vi "temp control global variables.vi"() -> ()   [LabVIEW 2016]
doc: "These are the global variables for the temperature control system including:\n\n1) The HP34401A globals\n2) The PID globals\n3) The Temp controller globals\n\nPaul K Dixon\nPhysics 350\nCSUSB Physics"
uses:
  typedefs/control parameters.ctl
  typedefs/scale control.ctl
panel:
  in  "Init controls":T1={"Function Picker (DCV)"=enum."DC Volts", "Range (T=Auto)"=TRUE, "Range"=10.0, "Resolution (T=Auto)"=TRUE, "Resolution"=0.001} {"Resolution" format="%.4f"; "Range" format="%.3f"}
  in  "init flag":bool
  in  "T cont exited":bool
  in  "exit T cont":bool
  in  "Scale Control":T2={"Full Scale"=FALSE, "Control Scale"=TRUE, "Settle Scale"=FALSE, "Zoom Out"=FALSE, "Zoom In"=FALSE}
  out "settled":bool
  in  "Control Parameters":T3={"Setpoint"=30.0, "Control bandwidth"=4.0, "Settle bandwidth"=1.0, "Integral time"=30.0, "Int\non"=TRUE, "Derivative time"=0.5, "Der\non"=TRUE, "Settle time"=30.0} {"Settle time" format="%.2f"; "Derivative time" format="%.2f"; "Integral time" format="%.2f"; "Settle bandwidth" format="%.2f"; "Control bandwidth" format="%.2f"; "Setpoint" format="%.2f"}
  in  "Reset PID (auto clear)":bool
  # "Temp Chart Global Variables"
  # "PID Global Variables"
  # "Simple HP34401 Driver Global Variables"
  # "Autorange"
  # "Use This ---->"
  # "Even with specific\nranging, autores is\nthe best way to go."
  # "Auto-Select"
  # "Use This ---->"
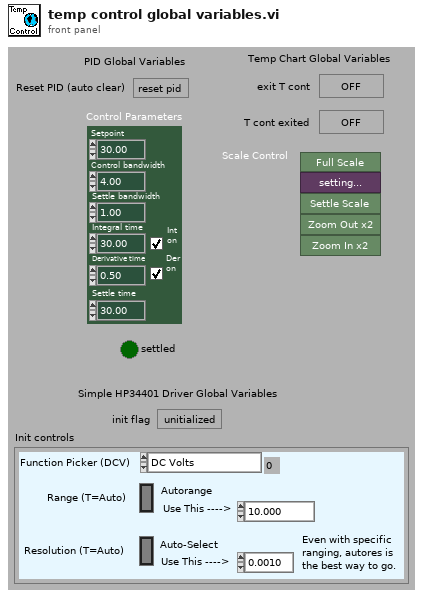
[diagram p1: front panel]
types:
  T1 = cluster{"Function Picker (DCV)":enum16{"DC Volts", "AC Volts", "DC Current", "AC Current", "Resistance", "Four Wire Resistance", "Frequency", "Period", "Continuity", "Diode Test"}, "Range (T=Auto)":bool, "Range":dbl, "Resolution (T=Auto)":bool, "Resolution":dbl}
  T2 = typedef "scale control.ctl" = cluster{"Full Scale":bool, "Control Scale":bool, "Settle Scale":bool, "Zoom Out":bool, "Zoom In":bool}
  T3 = typedef "control parameters.ctl" = cluster{"Setpoint":dbl, "Control bandwidth":dbl, "Settle bandwidth":dbl, "Integral time":dbl, "Int\non":bool, "Derivative time":dbl, "Der\non":bool, "Settle time":dbl}
diagram:
